vi "Check Step is Done.vi"(8 "error in (no error)":errorcluster, 11 "Stand in":refnum<class "Stand.lvclass">) -> (0 "error out":errorcluster, 3 "Stand out":refnum<class "Stand.lvclass">)   [LabVIEW 2019, in "Stand.lvclass"]
uses:
  Stand.lvclass
  Stand.lvclass/Stand.ctl
  AI_class/AI.lvclass/AI.ctl
  AnalogComparator_class/AnalogComparator.lvclass/AnalogComparator.ctl
  TypeDef/ExecuteStepState.ctl
  1310047f-972f-4ee0-907f-240588ea95d0.vi
  98531ce8-0a05-42df-884b-e0001e423214.vi
  AnalogComparator_class/GetStatus.vi
  Global/Global Constant.vi
  AI_class/AI.lvclass
panel:
  in  "init":bool
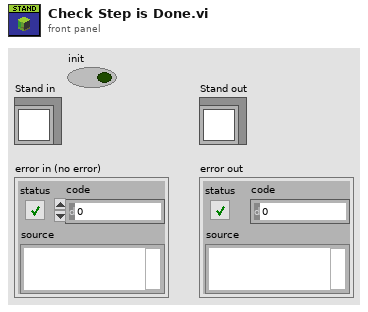
[diagram p1: front panel]
types:
  T1 = typedef "SP_TYPE.ctl" = enum16{"ERROR", "ZIRO", "BASE", "SP"}
  T2 = typedef "AI_Data.ctl" = cluster{"Stat Data":T3, "OutOfRangeMax":bool, "OutOfRangeMin":bool, "HIHI":bool, "HI":bool, "LO":bool, "LOLO":bool}
  T3 = typedef "AI Statistics Data.ctl" = cluster{"raw mean":dbl, "scl mean":dbl, "raw mean 1Hz":dbl, "scl mean 1Hz":dbl}
  T4 = typedef "ExecuteStepState.ctl" = enum16{"Init", "Set: Backpressure ", "Preload: HI", "Set: HI", "Maintenance: HI", "Down: Pressure", "BLOCK"}
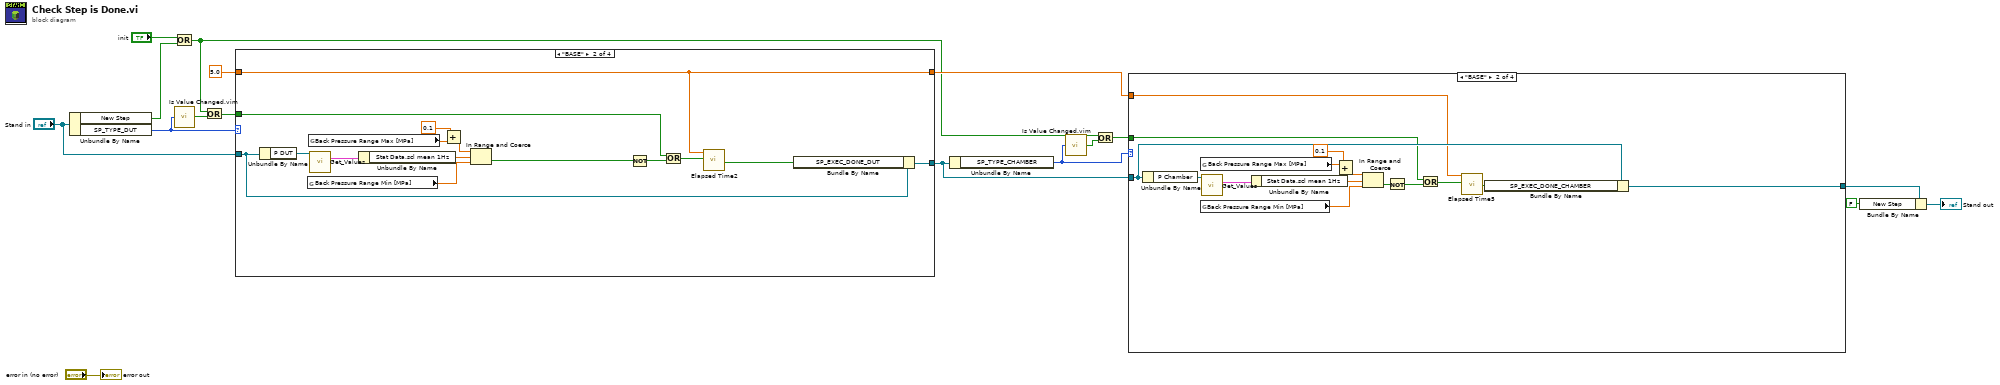
[diagram p0: block diagram]
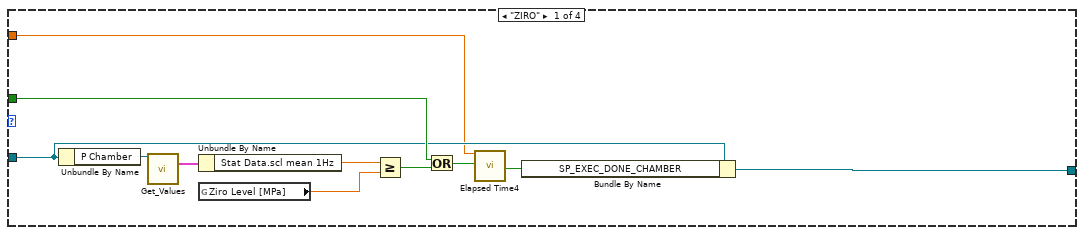
[diagram p2: hidden frame]
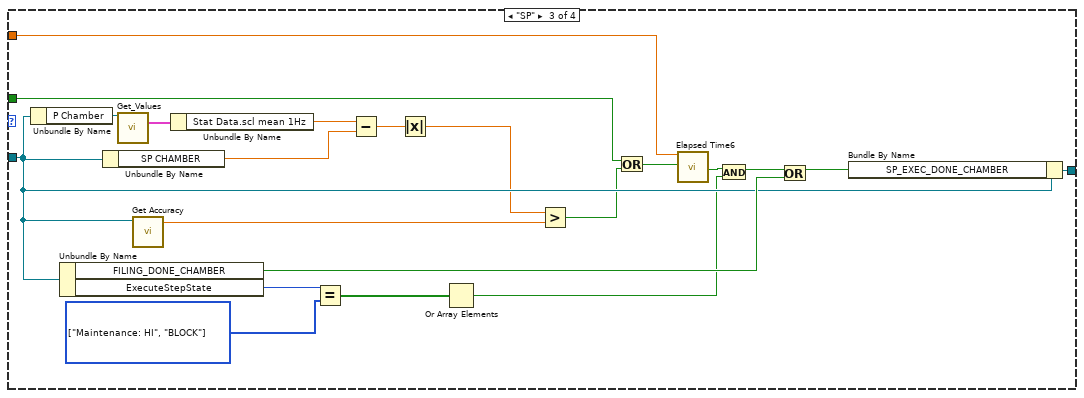
[diagram p3: hidden frame]
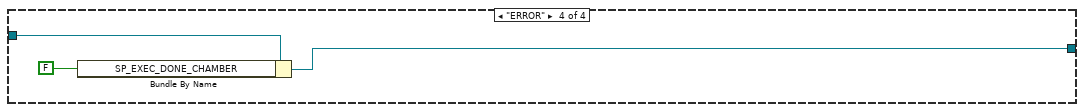
[diagram p4: hidden frame]
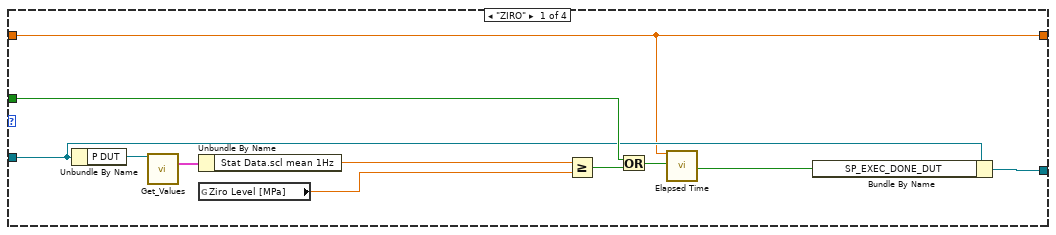
[diagram p5: hidden frame]
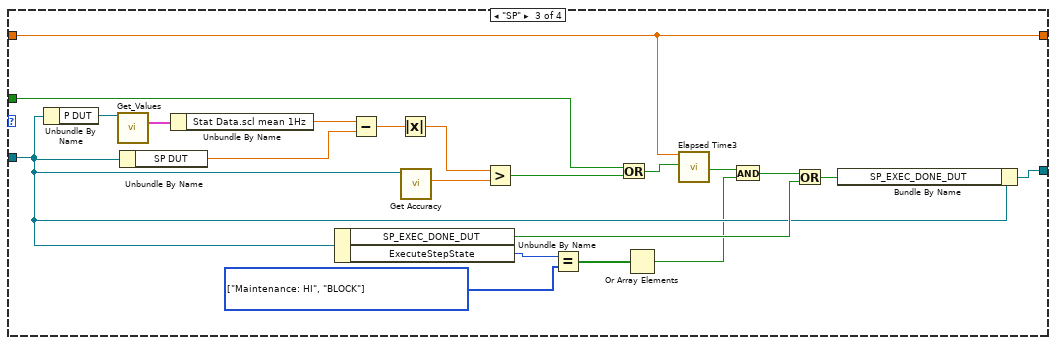
[diagram p6: hidden frame]
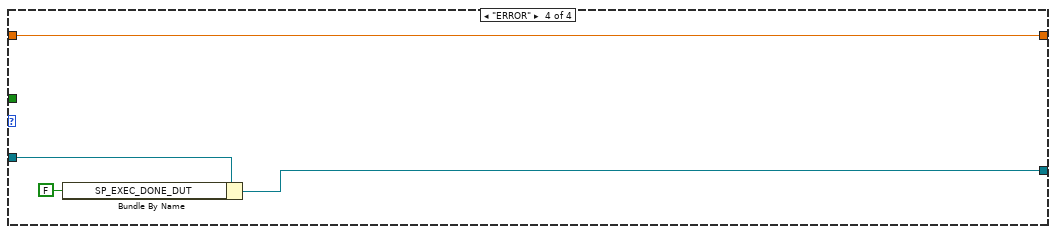
[diagram p7: hidden frame]
diagram:
  n1 = Unbundle By Name("Stand in") -> ("New Step"=w3:bool, "SP_TYPE_DUT"=w15:T1)
  n2 = Or(x="init", y=w3) -> (x .or. y?=w4:bool)
  n3 = call "Is Value Changed.vim"("value"=w15) -> ("changed or first call?"=w14:bool)
  n4 = Or(x=w4, y=w14) -> (x .or. y?=w13:bool)
  n5 = case shown="\"BASE\"" w15 {
    tunnel: "Stand in" -> [w20 w36 w48 w67]
    tunnel: [w19 w35 w60 w66] -> w9
    tunnel: w13 -> [w21 w34 w45 _]
    tunnel: 5.0 ("Time Target (s)") -> [w18 w31 w53 w65]
    tunnel: [w18 w31 w53 w65] -> w5
    frame "ZIRO" {
      n6 = Unbundle By Name(w20) -> ("P DUT"=w26:refnum<class "AI.lvclass">)
      n7 = call "Get_Values.vi"("reference in"=w26) -> ("Data"=w28:T2)  [unwired: 14 in]
      n8 = Unbundle By Name(w28) -> ("Stat Data.scl mean 1Hz"=w27:dbl)
      n9 = global read "Global Constant.vi" "Ziro Level [MPa]"() -> (w25:dbl)
      n10 = Greater Or Equal?(x=w27, y=w25) -> (x >= y?=w24:bool)
      n11 = Or(x=w21, y=w24) -> (x .or. y?=w23:bool)
      n12 = call "Elapsed Time"("Time Target (s)"=w18, "Reset"=w23) -> ("Time has Elapsed"=w22:bool)  [unwired: 10 in, 7 out]
      n13 = Bundle By Name(cluster=w20, "SP_EXEC_DONE_DUT"=w22) -> (w19:refnum<class "Stand.lvclass">)
    }
    frame "BASE" {
      n14 = Unbundle By Name(w36) -> ("P DUT"=w41:refnum<class "AI.lvclass">)
      n15 = global read "Global Constant.vi" "Back Pressure Range Min [MPa]"() -> (w43:dbl)
      n16 = global read "Global Constant.vi" "Back Pressure Range Max [MPa]"() -> (w42:dbl)
      n17 = call "Get_Values.vi"("reference in"=w41) -> ("Data"=w39:T2)  [unwired: 14 in]
      n18 = Unbundle By Name(w39) -> ("Stat Data.scl mean 1Hz"=w40:dbl)
      n19 = Add(x=0.1, y=w42) -> (x+y=w30:dbl)
      n20 = In Range and Coerce(upper limit=w30, x=w40, lower limit=w43) -> (In Range?=w33:bool)  [unwired: 1 out]
      n21 = Not(x=w33) -> (.not. x?=w32:bool)
      n22 = Or(x=w34, y=w32) -> (x .or. y?=w38:bool)
      n23 = call "Elapsed Time2"("Time Target (s)"=w31, "Reset"=w38) -> ("Time has Elapsed"=w37:bool)  [unwired: 10 in, 7 out]
      n24 = Bundle By Name(cluster=w36, "SP_EXEC_DONE_DUT"=w37) -> (w35:refnum<class "Stand.lvclass">)
    }
    frame "SP" {
      w52 = T4[] [enum."Maintenance: HI", enum."BLOCK"] items=["Init", "Set: Backpressure ", "Preload: HI", "Set: HI", "Maintenance: HI", "Down: Pressure", "BLOCK"] ("y")
      n25 = Unbundle By Name(w48) -> ("P DUT"=w64:refnum<class "AI.lvclass">)
      n26 = call "Get_Values.vi"("reference in"=w64) -> ("Data"=w63:T2)  [unwired: 14 in]
      n27 = Unbundle By Name(w48) -> ("SP DUT"=w57:dbl)
      n28 = Unbundle By Name(w63) -> ("Stat Data.scl mean 1Hz"=w58:dbl)
      n29 = Unbundle By Name(w48) -> ("SP_EXEC_DONE_DUT"=w54:bool, "ExecuteStepState"=w51:T4)
      n30 = Subtract(x=w58, y=w57) -> (x-y=w59:dbl)
      n31 = Absolute Value(x=w59) -> (abs(x)=w47:dbl)
      n32 = call "Get Accuracy.vi"("Stand in"=w48) -> ("Accuracy [MPa]"=w46:dbl)  [unwired: 10 in]
      n33 = Greater?(x=w47, y=w46) -> (0:w56:bool)
      n34 = Equal?(x=w51, y=w52) -> (x = y?=w49:bool[])
      n35 = Or(x=w45, y=w56) -> (x .or. y?=w62:bool)
      n36 = Or Array Elements(Boolean array=w49) -> (logical OR=w44:bool)
      n37 = call "Elapsed Time3"("Time Target (s)"=w53, "Reset"=w62) -> ("Time has Elapsed"=w61:bool)  [unwired: 10 in, 7 out]
      n38 = And(x=w61, y=w44) -> (x .and. y?=w50:bool)
      n39 = Or(x=w50, y=w54) -> (x .or. y?=w55:bool)
      n40 = Bundle By Name(cluster=w48, "SP_EXEC_DONE_DUT"=w55) -> (w60:refnum<class "Stand.lvclass">)
    }
    frame "ERROR" {
      n41 = Bundle By Name(cluster=w67, "SP_EXEC_DONE_DUT"=FALSE) -> (w66:refnum<class "Stand.lvclass">)
    }
  }
  n42 = Unbundle By Name(w9) -> ("SP_TYPE_CHAMBER"=w10:T1)
  n43 = call "Is Value Changed.vim"("value"=w10) -> ("changed or first call?"=w11:bool)
  n44 = Or(x=w4, y=w11) -> (x .or. y?=w12:bool)
  n45 = case shown="\"BASE\"" w10 {
    tunnel: w9 -> [w71 w87 w98 w117]
    tunnel: [w70 w86 w111 w116] -> w8
    tunnel: w12 -> [w72 w85 w110 _]
    tunnel: w5 -> [w69 w82 w109 _]
    frame "ZIRO" {
      n46 = Unbundle By Name(w71) -> ("P Chamber"=w77:refnum<class "AI.lvclass">)
      n47 = call "Get_Values.vi"("reference in"=w77) -> ("Data"=w79:T2)  [unwired: 14 in]
      n48 = Unbundle By Name(w79) -> ("Stat Data.scl mean 1Hz"=w78:dbl)
      n49 = global read "Global Constant.vi" "Ziro Level [MPa]"() -> (w76:dbl)
      n50 = Greater Or Equal?(x=w78, y=w76) -> (x >= y?=w75:bool)
      n51 = Or(x=w72, y=w75) -> (x .or. y?=w74:bool)
      n52 = call "Elapsed Time4"("Time Target (s)"=w69, "Reset"=w74) -> ("Time has Elapsed"=w73:bool)  [unwired: 10 in, 7 out]
      n53 = Bundle By Name(cluster=w71, "SP_EXEC_DONE_CHAMBER"=w73) -> (w70:refnum<class "Stand.lvclass">)
    }
    frame "BASE" {
      n54 = Unbundle By Name(w87) -> ("P Chamber"=w92:refnum<class "AI.lvclass">)
      n55 = global read "Global Constant.vi" "Back Pressure Range Min [MPa]"() -> (w94:dbl)
      n56 = global read "Global Constant.vi" "Back Pressure Range Max [MPa]"() -> (w93:dbl)
      n57 = call "Get_Values.vi"("reference in"=w92) -> ("Data"=w90:T2)  [unwired: 14 in]
      n58 = Unbundle By Name(w90) -> ("Stat Data.scl mean 1Hz"=w91:dbl)
      n59 = Add(x=w93, y=0.1) -> (x+y=w81:dbl)
      n60 = In Range and Coerce(upper limit=w81, x=w91, lower limit=w94) -> (In Range?=w84:bool)  [unwired: 1 out]
      n61 = Not(x=w84) -> (.not. x?=w83:bool)
      n62 = Or(x=w85, y=w83) -> (x .or. y?=w89:bool)
      n63 = call "Elapsed Time5"("Time Target (s)"=w82, "Reset"=w89) -> ("Time has Elapsed"=w88:bool)  [unwired: 10 in, 7 out]
      n64 = Bundle By Name(cluster=w87, "SP_EXEC_DONE_CHAMBER"=w88) -> (w86:refnum<class "Stand.lvclass">)
    }
    frame "SP" {
      w103 = T4[] [enum."Maintenance: HI", enum."BLOCK"] items=["Init", "Set: Backpressure ", "Preload: HI", "Set: HI", "Maintenance: HI", "Down: Pressure", "BLOCK"] ("y")
      n65 = Unbundle By Name(w98) -> ("P Chamber"=w115:refnum<class "AI.lvclass">)
      n66 = Unbundle By Name(w98) -> ("FILING_DONE_CHAMBER"=w102:bool, "ExecuteStepState"=w104:T4)
      n67 = Unbundle By Name(w98) -> ("SP CHAMBER"=w106:dbl)
      n68 = call "Get_Values.vi"("reference in"=w115) -> ("Data"=w114:T2)  [unwired: 14 in]
      n69 = call "Get Accuracy.vi"("Stand in"=w98) -> ("Accuracy [MPa]"=w99:dbl)  [unwired: 10 in]
      n70 = Unbundle By Name(w114) -> ("Stat Data.scl mean 1Hz"=w107:dbl)
      n71 = Equal?(x=w104, y=w103) -> (x = y?=w100:bool[])
      n72 = Subtract(x=w107, y=w106) -> (x-y=w108:dbl)
      n73 = Absolute Value(x=w108) -> (abs(x)=w97:dbl)
      n74 = Or Array Elements(Boolean array=w100) -> (logical OR=w95:bool)
      n75 = Greater?(x=w97, y=w99) -> (0:w96:bool)
      n76 = Or(x=w110, y=w96) -> (x .or. y?=w113:bool)
      n77 = call "Elapsed Time6"("Time Target (s)"=w109, "Reset"=w113) -> ("Time has Elapsed"=w112:bool)  [unwired: 10 in, 7 out]
      n78 = And(x=w112, y=w95) -> (x .and. y?=w101:bool)
      n79 = Or(x=w101, y=w102) -> (x .or. y?=w105:bool)
      n80 = Bundle By Name(cluster=w98, "SP_EXEC_DONE_CHAMBER"=w105) -> (w111:refnum<class "Stand.lvclass">)
    }
    frame "ERROR" {
      n81 = Bundle By Name(cluster=w117, "SP_EXEC_DONE_CHAMBER"=FALSE ("SP_EXEC_DONE_DUT")) -> (w116:refnum<class "Stand.lvclass">)
    }
  }
  n82 = Bundle By Name(cluster=w8, "New Step"=FALSE ("Data.New Step")) -> (→"Stand out":refnum<class "Stand.lvclass">)
  "error out" <- "error in (no error)"
